vi "Motion@GoPallet(SingleAxis)__Parameter.vi"(1 "ParamterIn":string) -> (0 "ParamterOut":string)   [LabVIEW 2020]
panel:
  in  "HeadNm":string(combo)
  in  "Offset":string(combo)
  in  "Head":string(combo)
  in  "AXIS":string(combo)
  in  "PointName":string(combo)
  in  "Speed":string(combo)
  in  "MotorName":string(combo)
  in  "Confirm":bool
  # "Motion@GoPallet(SingleAxis) $Motor,$Speed,$Point(@AXIS#Head&Offset)\nExample:  $Point@XY will move XY only\n               $Point@XYZ(5) will move XYZ and Z will replace by 5"
  # "@"
  # "["
  # "]"
  # "#"
  # "&"
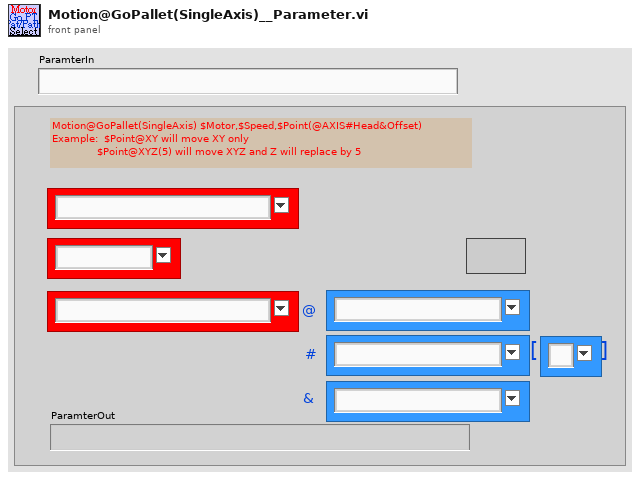
[diagram p1: front panel]
types:
  T1 = enum16{"Get", "UpdatePointS", "Init", "UpdateIndex", "GetCurrent&Index+1", "GetWithIndex", "ChkLast", "GetCurrent"}
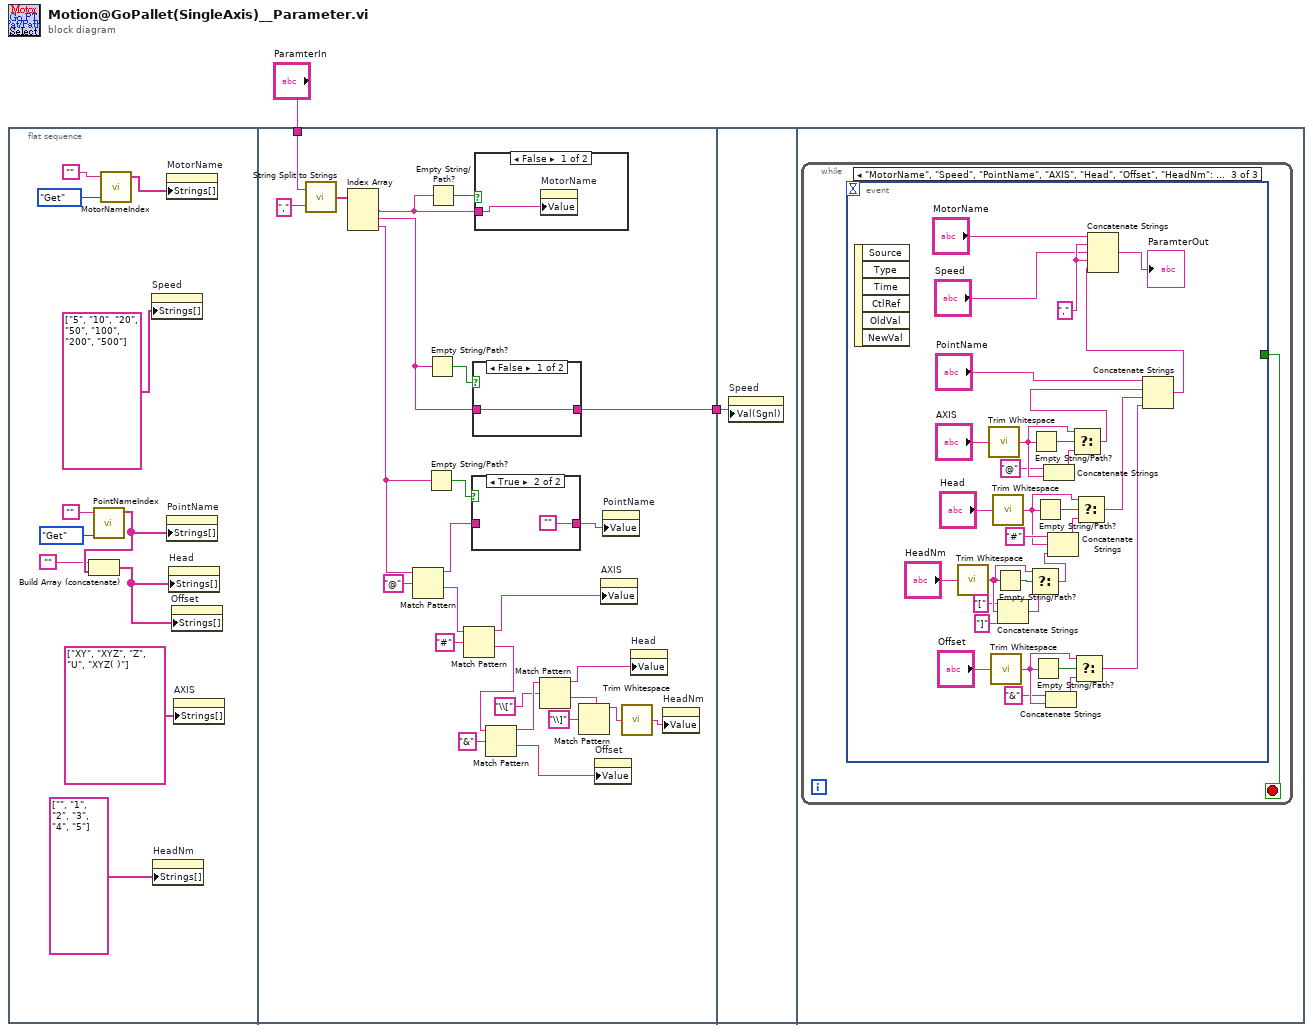
[diagram p0: block diagram]
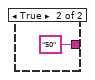
[diagram p3: hidden frame]
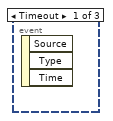
[diagram p5: hidden frame]
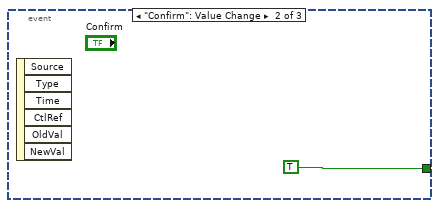
[diagram p6: hidden frame]
diagram:
  n1 = flat-sequence {
    tunnel: "ParamterIn" -> [w35]
    tunnel: [w31] -> w1
    tunnel: w1 -> [w45]
    frame #0 {
      n2 = call "PointNameIndex.vi"("OP"=T1."Get", "PointName"="") -> ("PointNameList"=w6:string[])  [unwired: 4 in, 5 out]
      n3 = Build Array (concatenate)("", w6) -> (w5:string[])
      n4 = call "MotorNameIndex.vi"("OP"=enum16{"Get", "Update", "Init"}."Get", "MotorName"="") -> ("MotorList"=w11:string[])  [unwired: 1 in, 2 out]
      n5 = property on="Speed" class="CmbBox"("Strings[]"=string[] ["5", "10", "20", "50", "100", "200", "500"] ("Strings []")) -> ()  [unwired: 2 in, 2 out]
      n6 = property on="HeadNm" class="CmbBox"("Strings[]"=string[] ["", "1", "2", "3", "4", "5"] ("Strings []")) -> ()  [unwired: 2 in, 2 out]
      n7 = property on="MotorName" class="CmbBox"("Strings[]"=w11) -> ()  [unwired: 2 in, 2 out]
      n8 = property on="PointName" class="CmbBox"("Strings[]"=w6) -> ()  [unwired: 2 in, 2 out]
      n9 = property on="Head" class="CmbBox"("Strings[]"=w5) -> ()  [unwired: 2 in, 2 out]
      n10 = property on="Offset" class="CmbBox"("Strings[]"=w5) -> ()  [unwired: 2 in, 2 out]
      n11 = property on="AXIS" class="CmbBox"("Strings[]"=string[] ["XY", "XYZ", "Z", "U", "XYZ( )"] ("Strings []")) -> ()  [unwired: 2 in, 2 out]
    }
    frame #1 {
      n12 = call "String Split to Strings.vi"("search string/char (-)"=",", "String"=w35) -> ("Array"=w37:string[])
      n13 = Index Array(array=w37) -> (element #1=w34:string, element #2=w33:string, element #3=w29:string)  [unwired: 3 in]
      n14 = Match Pattern(string=w29, regular expression="@") -> (before substring=w27:string, after substring=w25:string)  [unwired: 1 in, 2 out]
      n15 = Empty String/Path?(string/path=w29) -> (empty?=w32:bool)
      n16 = Empty String/Path?(string/path=w33) -> (empty?=w38:bool)
      n17 = Empty String/Path?(string/path=w34) -> (empty?=w39:bool)
      n18 = Match Pattern(string=w25, regular expression="#") -> (before substring=w24:string, after substring=w22:string)  [unwired: 1 in, 2 out]
      n19 = case shown="True" w32 {
        tunnel: [w40 ""] -> w30
        tunnel: w27 -> [w40 _]
        frame False {
        }
        frame True {
        }
      }
      n20 = case shown="False" w38 {
        tunnel: [w42 "50" ("ParamterIn")] -> w31
        tunnel: w33 -> [w42 _]
        frame False {
        }
        frame True {
        }
      }
      n21 = case shown="False" w39 {
        tunnel: w34 -> [w44 _]
        frame False {
          n22 = property on="MotorName" class="CmbBox"("Value"=w44) -> ()  [unwired: 2 in, 2 out]
        }
        frame True {
        }
      }
      n23 = Match Pattern(string=w22, regular expression="&") -> (before substring=w20:string, after substring=w21:string)  [unwired: 1 in, 2 out]
      n24 = Match Pattern(string=w20, regular expression="\\[") -> (before substring=w16:string, after substring=w18:string)  [unwired: 1 in, 2 out]
      n25 = Match Pattern(string=w18, regular expression="\\]") -> (before substring=w14:string)  [unwired: 1 in, 3 out]
      n26 = property on="Offset" class="CmbBox"("Value"=w21) -> ()  [unwired: 2 in, 2 out]
      n27 = property on="AXIS" class="CmbBox"("Value"=w24) -> ()  [unwired: 2 in, 2 out]
      n28 = property on="PointName" class="CmbBox"("Value"=w30) -> ()  [unwired: 2 in, 2 out]
      n29 = call <vilib>:"Trim Whitespace.vi"("string"=w14) -> ("trimmed string"=w15:string)  [unwired: 1 in]
      n30 = property on="Head" class="CmbBox"("Value"=w16) -> ()  [unwired: 2 in, 2 out]
      n31 = property on="HeadNm" class="CmbBox"("Value"=w15) -> ()  [unwired: 2 in, 2 out]
    }
    frame #2 {
      n32 = property on="Speed" class="CmbBox"("Val(Sgnl)"=w45) -> ()  [unwired: 2 in, 2 out]
    }
    frame #3 {
      n33 = while {
        stop <- w46 stop-if-true
        n34 = event shown="[2] \"MotorName\", \"Speed\", \"PointName\", \"AXIS\", \"Head\", \"Offset\", \"HeadNm\": Value Change" {
          selector: _ -> [_ _ _]
          dyn-events: _ -> [_ _ _]
          timeout: _ -> [_ _ _]
          tunnel: [_ TRUE _] -> w46
          event Timeout {
            n35 = event-data() -> ()  [unwired: 1 in, 3 out]
          }
          event "Confirm": Value Change {
            n36 = event-data() -> ()  [unwired: 1 in, 6 out]
          }
          event "MotorName", "Speed", "PointName", "AXIS", "Head", "Offset", "HeadNm": Value Change {
            w76 = "," ("string")
            n37 = event-data() -> ()  [unwired: 1 in, 6 out]
            n38 = call <vilib>:"Trim Whitespace.vi"("string"="HeadNm") -> ("trimmed string"=w52:string)  [unwired: 1 in]
            n39 = call <vilib>:"Trim Whitespace.vi"("string"="AXIS") -> ("trimmed string"=w71:string)  [unwired: 1 in]
            n40 = call <vilib>:"Trim Whitespace.vi"("string"="Offset") -> ("trimmed string"=w58:string)  [unwired: 1 in]
            n41 = call <vilib>:"Trim Whitespace.vi"("string"="Head") -> ("trimmed string"=w65:string)  [unwired: 1 in]
            n42 = Empty String/Path?(string/path=w52) -> (empty?=w53:bool)
            n43 = Concatenate Strings("[" ("string"), w52, "]" ("string")) -> (w49:string)
            n44 = Select(t=w52, s=w53, f=w49) -> (s? t:f=w48:string)
            n45 = Empty String/Path?(string/path=w71) -> (empty?=w73:bool)
            n46 = Empty String/Path?(string/path=w58) -> (empty?=w60:bool)
            n47 = Empty String/Path?(string/path=w65) -> (empty?=w63:bool)
            n48 = Concatenate Strings("@" ("string"), w71) -> (w72:string)
            n49 = Concatenate Strings("&" ("string"), w58) -> (w59:string)
            n50 = Concatenate Strings("#" ("string"), w65, w48) -> (w64:string)
            n51 = Select(t=w71, s=w73, f=w72) -> (s? t:f=w68:string)
            n52 = Select(t=w58, s=w60, f=w59) -> (s? t:f=w55:string)
            n53 = Select(t=w65, s=w63, f=w64) -> (s? t:f=w56:string)
            n54 = Concatenate Strings("PointName", w68, w56, w55) -> (w67:string)
            n55 = Concatenate Strings("MotorName", w76, "Speed", w76, w67) -> (→"ParamterOut":string)
          }
        }
      }
    }
  }
